vi "TransformObjectPosition_Objects.vi"(4 "Pixel size Y":dbl, 6 "Image time":dbl, 8 "error in (no error)":errorcluster, 9 "Pixel size X":dbl, 10 "Objects":T1(array[cluster]) {"Aspect Ratio" format="%.2f"; "Orientation" format="%.2f"; "Area" format="%.2f"; "Object Center"."Y" format="%.2f"; "Object Center"."X" format="%.2f"}, 11 "Spacetime cluster":T2) -> (0 "error out":errorcluster, 1 "Focus out":dbl, 2 "Y out":dbl, 3 "X out":dbl)   [LabVIEW 2012]
panel:
  out "Y center":dbl(graph)
  out "X center":dbl(graph)
  out "X stage":dbl(graph)
  out "Y stage":dbl(graph)
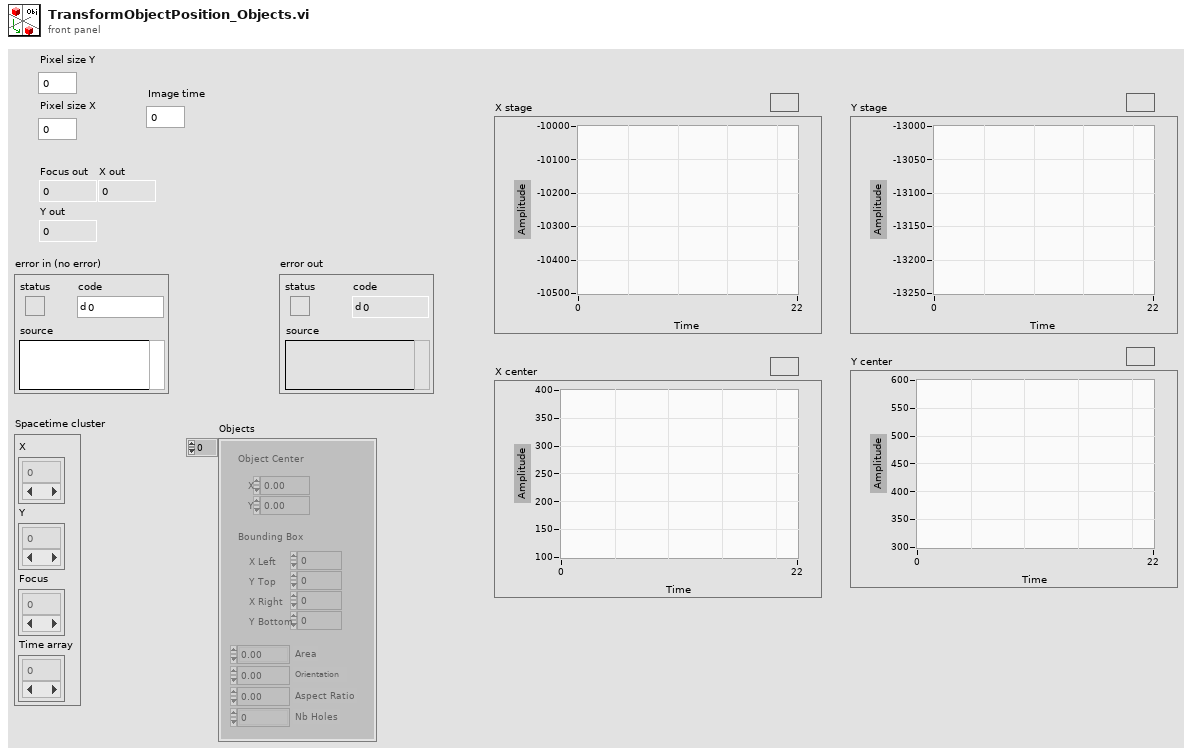
[diagram p1: front panel]
types:
  T1 = cluster{"Object Center":cluster{"X":sgl, "Y":sgl}, "Bounding Box":cluster{"X Left":i32, "Y Top":i32, "X Right":i32, "Y Bottom":i32}, "Area":sgl, "Orientation":sgl, "Aspect Ratio":sgl, "Nb Holes":i32}[]
  T2 = cluster{"X":dbl[], "Y":dbl[], "Focus":dbl[], "Time array":dbl[]}
  T3 = cluster{"Object Center":cluster{"X":sgl, "Y":sgl}, "Bounding Box":cluster{"X Left":i32, "Y Top":i32, "X Right":i32, "Y Bottom":i32}, "Area":sgl, "Orientation":sgl, "Aspect Ratio":sgl, "Nb Holes":i32}
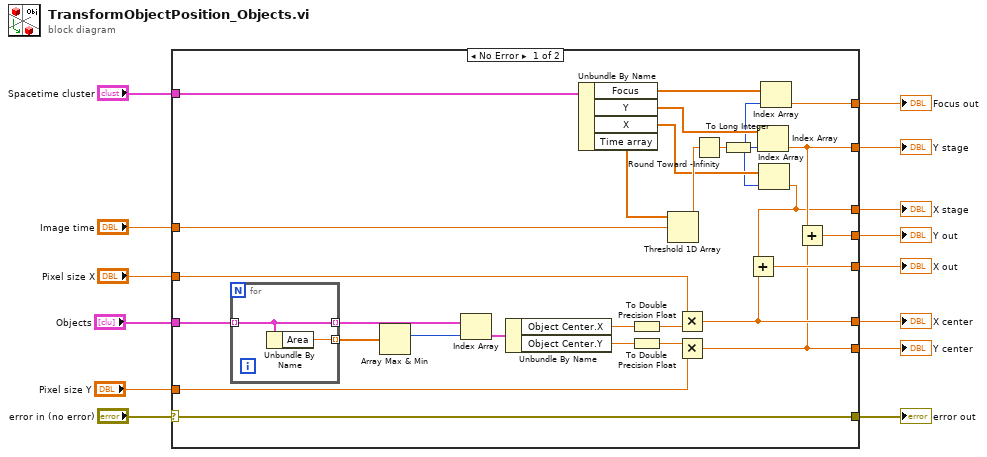
[diagram p0: block diagram]
diagram:
  n1 = case shown="No Error" "error in (no error)" {
    selector: "error in (no error)" -> [w37 w45]
    tunnel: [w37 w45] -> w13
    tunnel: "Objects" -> [w21 _]
    tunnel: "Pixel size X" -> [w41 _]
    tunnel: "Image time" -> [w40 _]
    tunnel: [w17 _] -> w10
    tunnel: [w39 _] -> w9
    tunnel: [w38 _] -> w8
    tunnel: "Spacetime cluster" -> [w36 _]
    tunnel: [w31 _] -> w6
    tunnel: [w29 _] -> w5
    tunnel: [w27 _] -> w4
    tunnel: [w26 _] -> w3
    tunnel: "Pixel size Y" -> [w24 _]
    frame No Error {
      n2 = for {
        tunnel: w21 -> [w43] mode=indexing
        tunnel: [w44] -> w19 mode=indexing
        tunnel: [w43] -> w20 mode=indexing
        n3 = Unbundle By Name(w43) -> ("Area"=w44:sgl)
      }
      n4 = Array Max & Min(array=w19) -> (max index (indices)=w18:i32)  [unwired: 3 out]
      n5 = Index Array(array=w20, index=w18) -> (element=w42:T3)
      n6 = Unbundle By Name(w42) -> ("Object Center.X"=w28:sgl, "Object Center.Y"=w25:sgl)
      n7 = Unbundle By Name(w36) -> ("Focus"=w16:dbl[], "Y"=w32:dbl[], "X"=w30:dbl[], "Time array"=w35:dbl[])
      n8 = To Double Precision Float(number=w28) -> (double precision float=w23:dbl)
      n9 = To Double Precision Float(number=w25) -> (double precision float=w22:dbl)
      n10 = Threshold 1D Array(2:w40, 3:w35) -> (0:w34:dbl)  [unwired: 1 in]
      n11 = Multiply(x=w41, y=w23) -> (x*y=w27:dbl)
      n12 = Multiply(x=w22, y=w24) -> (x*y=w26:dbl)
      n13 = Round Toward -Infinity(1:w34) -> (0:w33:dbl)
      n14 = To Long Integer(number=w33) -> (32bit integer=w15:i32)
      n15 = Index Array(array=w32, index=w15) -> (element=w31:dbl)
      n16 = Index Array(array=w30, index=w15) -> (element=w29:dbl)
      n17 = Add(x=w29, y=w27) -> (x+y=w38:dbl)
      n18 = Index Array(array=w16, index=w15) -> (element=w17:dbl)
      n19 = Add(x=w31, y=w26) -> (x+y=w39:dbl)
    }
    frame Error {
    }
  }
  "error out" <- w13
  "Focus out" <- w10
  "Y out" <- w9
  "X out" <- w8
  "Y stage" <- w6
  "X stage" <- w5
  "X center" <- w4
  "Y center" <- w3
